vi "Global Hint.vi"() -> ()   [LabVIEW 2014]
panel:
  out "Global Hint":dbl[][](array[numeric])
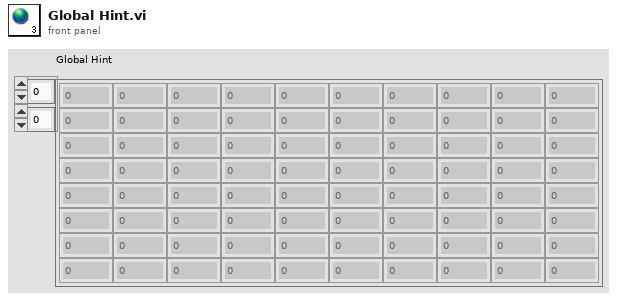
[diagram p1: front panel]
diagram:
